vi "G4SubTemplate_Simple_6x8x6_ReadProperty.vi"(8 "error in (no error)":errorcluster, 11 "reference in":refnum<class "G4SubTemplate_Simple_6x8x6.lvclass">) -> (0 "error out":errorcluster, 2 "property":dbl, 3 "reference out":refnum<class "G4SubTemplate_Simple_6x8x6.lvclass">)   [LabVIEW 2020]
uses:
  <resource>/Framework/Providers/Open_GDS/ClassProviders/Provider_EndevoGOOP400/Templates/G4SubTemplate_Simple_6x8x6/G4SubTemplate_Simple_6x8x6.lvclass
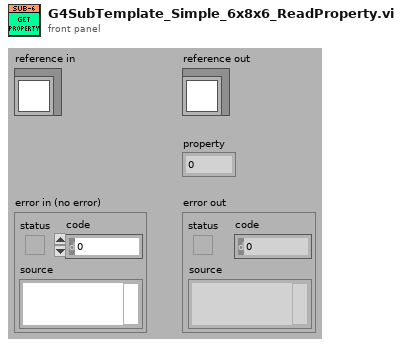
[diagram p1: front panel]
types:
  T1 = typedef "G4SubTemplate_Simple_6x8x6.lvclass/ObjectAttributes.ctl" = cluster{"Attribute1":dbl}
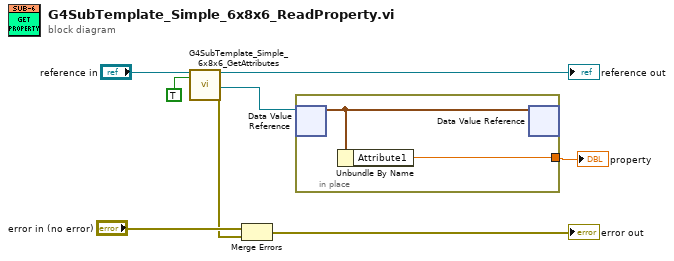
[diagram p0: block diagram]
diagram:
  n1 = call <resource>:"G4SubTemplate_Simple_6x8x6_GetAttributes.vi"("reference in"="reference in", "OnlyGetDvrReference(False)"=TRUE) -> ("reference out"=→"reference out":refnum<class "G4SubTemplate_Simple_6x8x6.lvclass">, "DataRef"=w2:refnum<data-value>, "error out"=w5:errorcluster)  [unwired: 14 in, 1 out]
  n2 = Merge Errors("error in (no error)", w5) -> (→"error out":errorcluster)
  n3 = in-place {
    in-place-border: [w10] -> w3
    n4 = in-place-dvr #1(w2) -> (w9:T1)  [unwired: 1 out]
    n5 = Unbundle By Name(w9) -> ("Attribute1"=w10:dbl)
    n6 = in-place-dvr #1(w9) -> ()  [unwired: 2 out]
  }
  "property" <- w3
